vi "Handle getAll.vi"(8 "error in (no error)":errorcluster, 11 "instrument.PPMS1 in":refnum<class "instrument.PPMS1.lvclass">) -> (0 "error out":errorcluster, 2 "getAll":variant, 3 "instrument.PPMS1 out":refnum<class "instrument.PPMS1.lvclass">)   [LabVIEW 2019, in "instrument.PPMS1.lvclass"]
uses:
  instrument.PPMS1.lvclass
  instrument.PPMS/instrument.PPMS.lvclass
  instrument.PPMS/Typedefs/PPMS.getAll--cluster.ctl
  C:/Users/patrick/Documents/GitHub/PPMS-Monitor-and-Control/lvsrc/instrument.PPMS/instrument.PPMS.lvclass
  C:/Program Files (x86)/National Instruments/LabVIEW 2019/user.lib/LevyLab/Levylab Instruments/Instrument Types/Cryostat/Instrument.Cryostat.lvclass
  C:/Program Files (x86)/National Instruments/LabVIEW 2019/user.lib/LevyLab/Levylab Instruments/SMOs/Instrument/Instrument.lvclass
  C:/Program Files (x86)/National Instruments/LabVIEW 2019/vi.lib/JKI/JKI SMO/SMO/SMO.lvclass
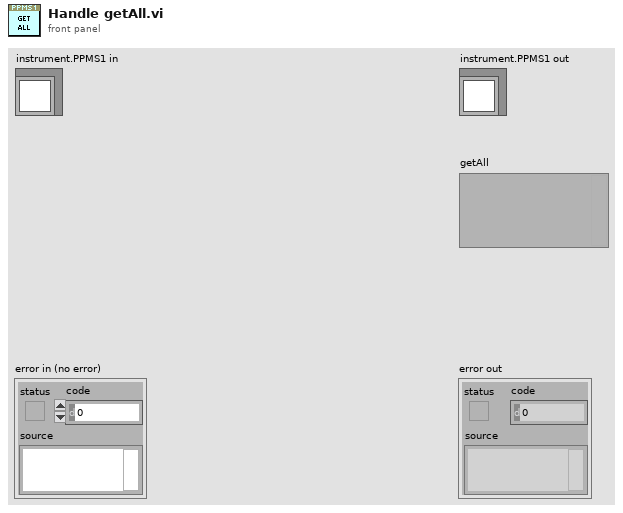
[diagram p1: front panel]
types:
  T1 = typedef "instrument.PPMS.lvclass/PPMS.getAll--cluster.ctl" = cluster{"Chamber Status":string, "Helium Level (%)":dbl, "Temperature (K)":dbl, "Temperature Status":string, "Magnetic Field (T)":dbl, "Magnet Status":string, "Position (°)":dbl}
  T2 = typedef "instrument.PPMS.lvclass/PPMS.Temperature Status--cluster.ctl" = cluster{"Temperature (K)":dbl, "Temperature Status":string}
  T3 = typedef "instrument.PPMS.lvclass/PPMS.Magnet Status--cluster.ctl" = cluster{"Field (T)":dbl, "Magnet Status":string}
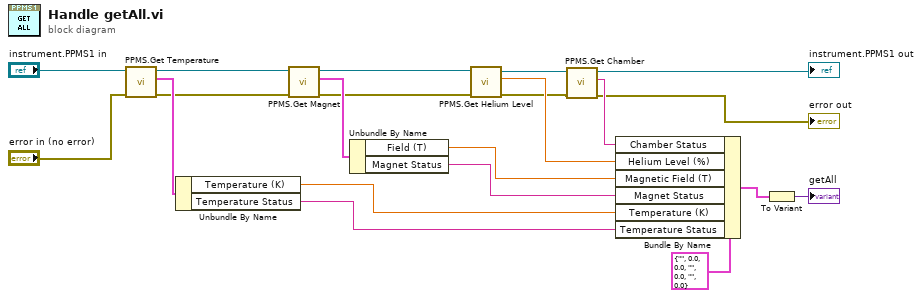
[diagram p0: block diagram]
diagram:
  n1 = call "PPMS.Get Temperature.vi"("error in (no error)"="error in (no error)", "instrument.PPMS"="instrument.PPMS1 in") -> ("error out"=w15:errorcluster, "Temperature Status"=w17:T2, "instrument.PPMS out"=w19:refnum<class "instrument.PPMS1.lvclass">)  [unwired: 7 in]
  n2 = Unbundle By Name(w17) -> ("Temperature (K)"=w11:dbl, "Temperature Status"=w10:string)
  n3 = call "PPMS.Get Magnet.vi"("error in (no error)"=w15, "instrument.PPMS"=w19) -> ("error out"=w14:errorcluster, "Magnet Status"=w16:T3, "instrument.PPMS out"=w18:refnum<class "instrument.PPMS1.lvclass">)  [unwired: 7 in]
  n4 = Unbundle By Name(w16) -> ("Field (T)"=w8:dbl, "Magnet Status"=w9:string)
  n5 = call "PPMS.Get Helium Level.vi"("error in (no error)"=w14, "instrument.PPMS"=w18) -> ("error out"=w4:errorcluster, "Helium Level (%)"=w7:dbl, "instrument.PPMS out"=w3:refnum<class "instrument.PPMS1.lvclass">)  [unwired: 7 in]
  n6 = call "PPMS.Get Chamber.vi"("error in (no error)"=w4, "instrument.PPMS"=w3) -> ("error out"=→"error out":errorcluster, "Status String"=w5:string, "instrument.PPMS out"=→"instrument.PPMS1 out":refnum<class "instrument.PPMS1.lvclass">)  [unwired: 7 in]
  n7 = Bundle By Name(cluster=T1 {"Chamber Status"="", "Helium Level (%)"=0.0, "Temperature (K)"=0.0, "Temperature Status"="", "Magnetic Field (T)"=0.0, "Magnet Status"="", "Position (°)"=0.0} ("getAll"), "Chamber Status"=w5, "Helium Level (%)"=w7, "Magnetic Field (T)"=w8, "Magnet Status"=w9, "Temperature (K)"=w11, "Temperature Status"=w10) -> (w20:T1)
  n8 = To Variant(anything=w20) -> (Variant=→"getAll":variant)
